vi "Save Capture Analyzer Measurement IQ Data.vi"(8 "error in (no error)":errorcluster, 9 "IQ File (\"file\")":string="file", 10 "Instance (1)":i32=1, 11 "VISA resource name":refnum<visa-resource-name>) -> (0 "error out":errorcluster, 3 "VISA resource name out":refnum<visa-resource-name>)   [LabVIEW 2020, in "Rohde&Schwarz CMXP GPRF.lvlib"]
doc: "Saves the I/Q data for the current step to the selected file.\n\nAttribute:\nRSCMXPGPRF_ATTR_CAPTURE_ANALYZER_MEASUREMENT_SAVE_IQ_FILE\n\nRemote-control command:\nCONFigure:GPRF:MEAS<i>:CANalyzer:IQFile"
uses:
  <instrlib>/Rohde&Schwarz CMXP GPRF/Rohde&Schwarz CMXP GPRF.lvlib
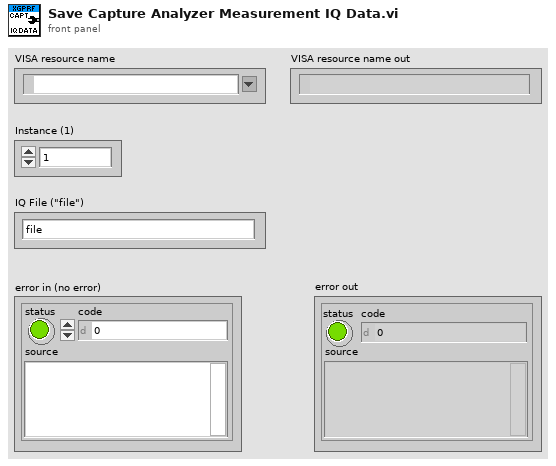
[diagram p1: front panel]
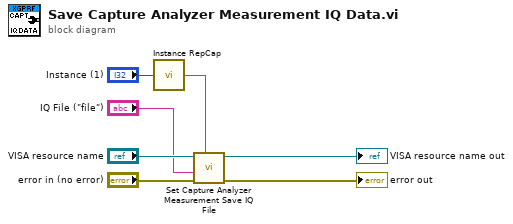
[diagram p0: block diagram]
diagram:
  n1 = call <instrlib>:"Instance RepCap.vi"("Instance in"="Instance (1)") -> ("Instance out"=w2:string)
  n2 = call "Set Capture Analyzer Measurement Save IQ File"("Repeated Capabilities"=w2, "error in (no error)"="error in (no error)", "Capture Analyzer Measurement Save IQ File ()"="IQ File (\"file\")", "instrument handle"="VISA resource name") -> ("error out"=→"error out":errorcluster, "instrument handle out"=→"VISA resource name out":refnum<visa-resource-name>)  [unwired: 6 in]
